vi "Filter State.vi"() -> ()   [LabVIEW 2023, in "Digikrom DK24x.lvlib"]
uses:
  Digikrom DK24x.lvlib
panel:
  in  "FILTER":u8=1 min=1 max=6 step=1
  # "DK24x does not have a command to query filter position\nWe will store it in this state variable instead."
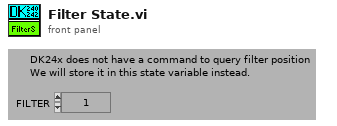
[diagram p1: front panel]
diagram:
